vi "ResizeFacade.vi"   [LabVIEW 2019, in "ExpandHorizontal.xctl"]
uses:
  ExpandHorizontal.xctl
types:
  T1 = typedef "LVRectTypeDef.ctl" = cluster{"Left":i16, "Top":i16, "Right":i16, "Bottom":i16}
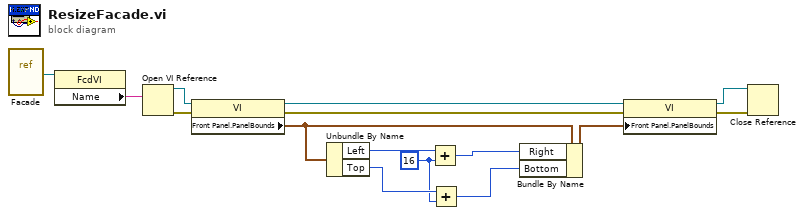
[diagram p0: block diagram]
diagram:
  w5 = i16 16 ("y")
  n1 = vi-ref "Facade.vi"() -> (w15:refnum<vi>)
  n2 = property class="FcdVI"(reference=w15) -> ("Name"=w14:string)  [unwired: 1 in, 2 out]
  n3 = Open VI Reference(vi path=w14) -> (vi reference=w3:refnum<vi>, error out=w4:errorcluster)  [unwired: 5 in]
  n4 = property class="VI"(reference=w3, error in=w4) -> (reference out=w13:refnum<vi>, error out=w12:errorcluster, "Front Panel.PanelBounds"=w10:T1)
  n5 = Unbundle By Name(w10) -> ("Left"=w7:i16, "Top"=w8:i16)
  n6 = Add(x=w7, y=w5) -> (x+y=w6:i16)
  n7 = Add(x=w8, y=w5) -> (x+y=w9:i16)
  n8 = Bundle By Name(cluster=w10, "Right"=w6, "Bottom"=w9) -> (w11:T1)
  n9 = property class="VI"(reference=w13, error in=w12, "Front Panel.PanelBounds"=w11) -> (reference out=w1:refnum<vi>, error out=w2:errorcluster)
  n10 = Close Reference(reference=w1, error in (no error)=w2) -> ()  [unwired: 1 out]
